vi "pythonTest.vi"() -> ()   [LabVIEW 2017]
panel:
  in  "stop":bool
  out "U16 Array Indicator":u16[](array[numeric])=[0, 1, 2, 3]
  out "U32 Indicator":u32=16 format="%x"
  in  "U16 Control":u16
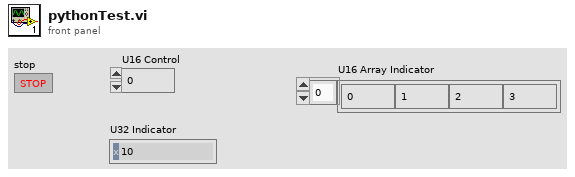
[diagram p1: front panel]
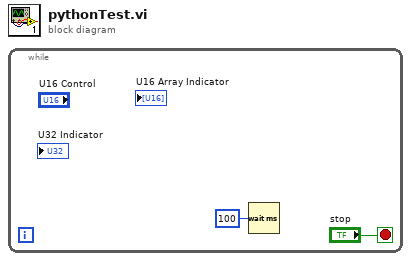
[diagram p0: block diagram]
diagram:
  n1 = while {
    stop <- "stop" stop-if-true
    n2 = Wait (ms)(milliseconds to wait=u32 100) -> ()  [unwired: 1 out]
  }
